vi "Heat2D_Form Y RHS.vi"(6 "step":i32, 7 "U(n+1/2)":dbl[][](array[numeric]), 8 "Boundary Condition":cluster{"type":T2, "Value":dbl[][]}[](array[cluster]) {"type" items=["Dirichlet", "Neumann"]}, 10 "Coefficients":T1) -> (1 "Y RHS out":dbl[][](array[numeric]), 2 "U down":dbl[](array[numeric]), 3 "U up":dbl[](array[numeric]))   [LabVIEW 2020, in "NI_PDE.lvlib"]
uses:
  <vilib>/gmath/NI_PDE.lvlib
  <vilib>/gmath/pde.llb/Common/PDE_BC Type.ctl
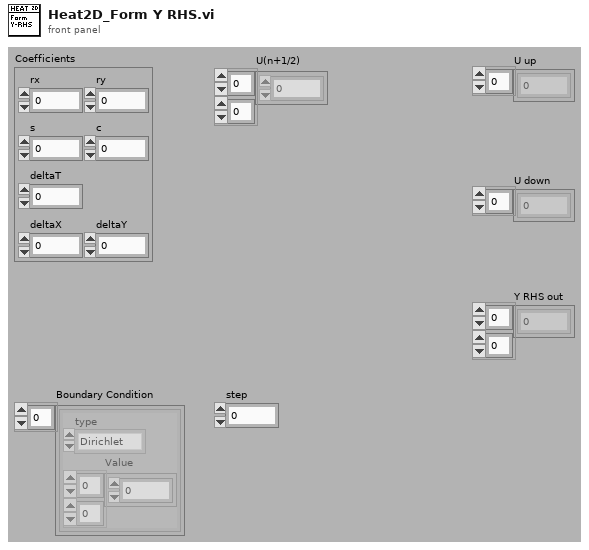
[diagram p1: front panel]
types:
  T1 = cluster{"rx":dbl, "ry":dbl, "s":dbl, "c":dbl, "deltaT":dbl, "deltaX":dbl, "deltaY":dbl}
  T2 = typedef "NI_PDE.lvlib/PDE_BC Type.ctl" = i32
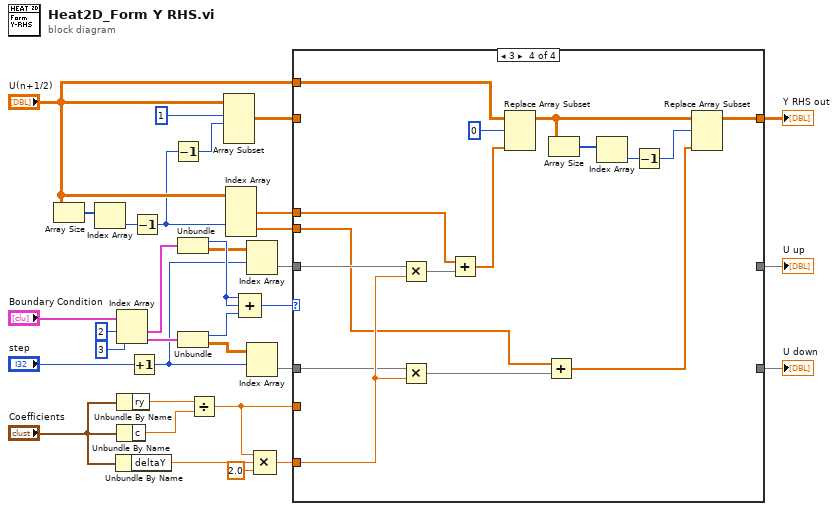
[diagram p0: block diagram]
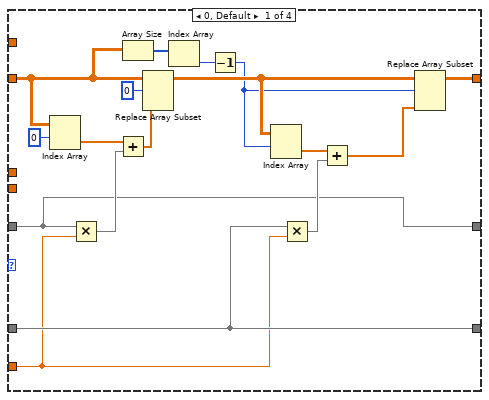
[diagram p2: hidden frame]
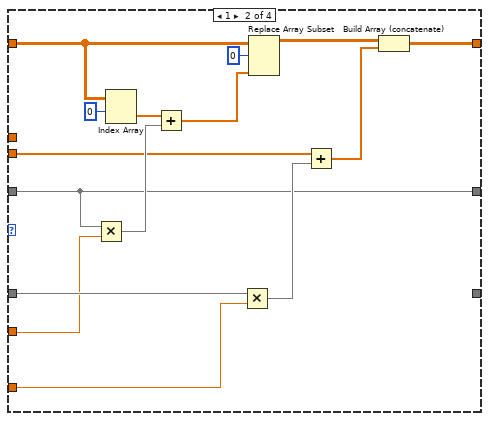
[diagram p3: hidden frame]
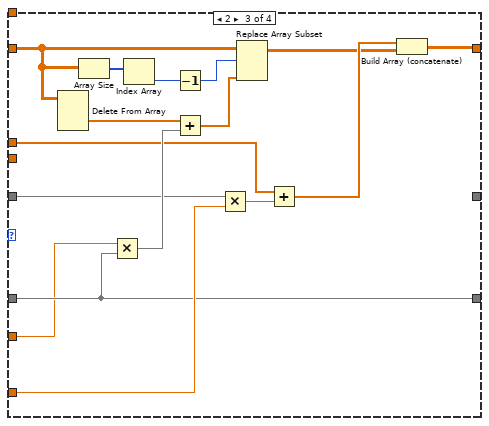
[diagram p4: hidden frame]
diagram:
  n1 = Array Size(array="U(n+1/2)") -> (size(s)=w8:i32[])
  n2 = Index Array(array=w8) -> (element=w6:i32)  [unwired: 1 in]
  n3 = Unbundle By Name("Coefficients") -> ("deltaY"=w17:dbl)
  n4 = Index Array(array="Boundary Condition", index #1=2 ("index"), index #2=3 ("index")) -> (element #1=w30:cluster{"type":T2, "Value":dbl[][]}, element #2=w29:cluster{"type":T2, "Value":dbl[][]})
  n5 = Unbundle By Name("Coefficients") -> ("ry"=w21:dbl)
  n6 = Unbundle By Name("Coefficients") -> ("c"=w20:dbl)
  n7 = Increment(x="step") -> (x+1=w11:i32)
  n8 = Decrement(x=w6) -> (x-1=w2:i32)
  n9 = Decrement(x=w2) -> (x-1=w1:i32)
  n10 = Unbundle(w30) -> ("type"=w28:T2, "Value"=w23:dbl[][])
  n11 = Unbundle(w29) -> ("type"=w27:T2, "Value"=w25:dbl[][])
  n12 = Divide(x=w21, y=w20) -> (x/y=w19:dbl)
  n13 = Array Subset(array="U(n+1/2)", index (row)=1 ("index"), length (row)=w1) -> (w4:dbl[][])  [unwired: 2 in]
  n14 = Index Array(array="U(n+1/2)", index (row) #2=w2) -> (element #1=w9:dbl[], element #2=w7:dbl[])  [unwired: 3 in]
  n15 = Compound Arithmetic op=ADD(w28, w28, w27) -> (w26:T2)
  n16 = Index Array(array=w23, index (row)=w11) -> (element=w22:dbl[])  [unwired: 1 in]
  n17 = Index Array(array=w25, index (row)=w11) -> (element=w24:dbl[])  [unwired: 1 in]
  n18 = Compound Arithmetic op=MULTIPLY(w19, w17, 2.0 ("value")) -> (w15:dbl)
  n19 = case shown="3" w26 {
    tunnel: w24 -> [w41 w61 w70 w94]
    tunnel: w22 -> [w36 w51 w78 w97]
    tunnel: w4 -> [w34 w65 w74 _]
    tunnel: w7 -> [_ w54 _ w91]
    tunnel: w9 -> [_ _ w75 w92]
    tunnel: w19 -> [w37 w60 w69 _]
    tunnel: [w39 w56 w66 w88] -> w14
    tunnel: w15 -> [_ w58 w77 w95]
    tunnel: [w41 _ w70 _] -> w13
    tunnel: [w36 w51 _ _] -> w12
    tunnel: "U(n+1/2)" -> [_ _ _ w82]
    frame 0, Default {
      n20 = Index Array(array=w34, index (row)=0) -> (element=w45:dbl[])  [unwired: 1 in]
      n21 = Multiply(x=w36, y=w37) -> (x*y=w44:dbl[])
      n22 = Add(x=w45, y=w44) -> (x+y=w43:dbl[])
      n23 = Array Size(array=w34) -> (size(s)=w50:i32[])
      n24 = Replace Array Subset(array=w34, new element=w43, index (row)=0) -> (w38:dbl[][])  [unwired: 1 in]
      n25 = Index Array(array=w50) -> (element=w49:i32)  [unwired: 1 in]
      n26 = Decrement(x=w49) -> (x-1=w35:i32)
      n27 = Index Array(array=w38, index (row)=w35) -> (element=w48:dbl[])  [unwired: 1 in]
      n28 = Multiply(x=w41, y=w37) -> (x*y=w46:dbl[])
      n29 = Add(x=w48, y=w46) -> (x+y=w47:dbl[])
      n30 = Replace Array Subset(array=w38, new element=w47, index (row)=w35) -> (w39:dbl[][])  [unwired: 1 in]
    }
    frame 1 {
      n31 = Multiply(x=w51, y=w60) -> (x*y=w62:dbl[])
      n32 = Index Array(array=w65, index (row)=0) -> (element=w64:dbl[])  [unwired: 1 in]
      n33 = Add(x=w64, y=w62) -> (x+y=w63:dbl[])
      n34 = Multiply(x=w61, y=w58) -> (x*y=w57:dbl[])
      n35 = Replace Array Subset(array=w65, new element=w63, index (row)=0) -> (w59:dbl[][])  [unwired: 1 in]
      n36 = Add(x=w54, y=w57) -> (x+y=w55:dbl[])
      n37 = Build Array (concatenate)(w59, w55) -> (w56:dbl[][])
    }
    frame 2 {
      n38 = Delete From Array(array=w74) -> (deleted portion=w81:dbl[])  [unwired: 3 in, 1 out]
      n39 = Array Size(array=w74) -> (size(s)=w73:i32[])
      n40 = Multiply(x=w69, y=w70) -> (x*y=w80:dbl[])
      n41 = Index Array(array=w73) -> (element=w72:i32)  [unwired: 1 in]
      n42 = Decrement(x=w72) -> (x-1=w71:i32)
      n43 = Add(x=w81, y=w80) -> (x+y=w79:dbl[])
      n44 = Multiply(x=w78, y=w77) -> (x*y=w76:dbl[])
      n45 = Replace Array Subset(array=w74, new element=w79, index (row)=w71) -> (w67:dbl[][])  [unwired: 1 in]
      n46 = Add(x=w75, y=w76) -> (x+y=w68:dbl[])
      n47 = Build Array (concatenate)(w68, w67) -> (w66:dbl[][])
    }
    frame 3 {
      n48 = Multiply(x=w97, y=w95) -> (x*y=w96:dbl[])
      n49 = Multiply(x=w94, y=w95) -> (x*y=w93:dbl[])
      n50 = Add(x=w92, y=w96) -> (x+y=w89:dbl[])
      n51 = Replace Array Subset(array=w82, new element=w89, index (row)=0) -> (w86:dbl[][])  [unwired: 1 in]
      n52 = Add(x=w91, y=w93) -> (x+y=w87:dbl[])
      n53 = Array Size(array=w86) -> (size(s)=w85:i32[])
      n54 = Index Array(array=w85) -> (element=w84:i32)  [unwired: 1 in]
      n55 = Decrement(x=w84) -> (x-1=w83:i32)
      n56 = Replace Array Subset(array=w86, new element=w87, index (row)=w83) -> (w88:dbl[][])  [unwired: 1 in]
    }
  }
  "Y RHS out" <- w14
  "U down" <- w13
  "U up" <- w12
